vi "Flywheel At Speed Check.vi"(11 "Shooter Speed Calibration":dbl) -> ()   [LabVIEW 2016]
uses:
  Global Variables/Sensor Data.vi
  Global Variables/Shooter Calibrations.vi
  Global Variables/Robot Status.vi
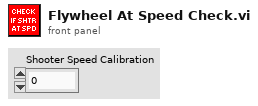
[diagram p1: front panel]
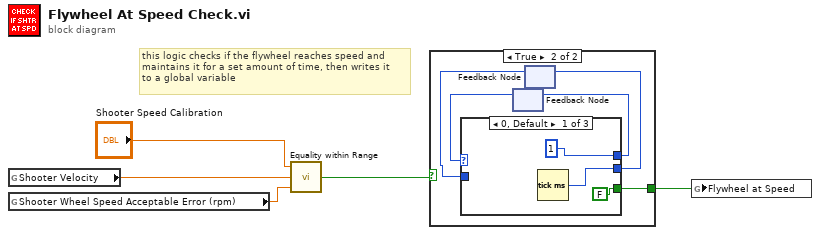
[diagram p0: block diagram]
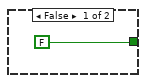
[diagram p2: hidden frame]
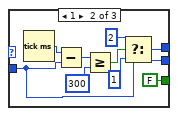
[diagram p3: hidden frame]
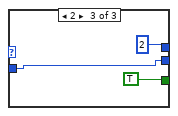
[diagram p4: hidden frame]
diagram:
  # "this logic checks if the flywheel reaches speed and\nmaintains it for a set amount of time, then writes it\nto a global variable"
  n1 = global read "Sensor Data.vi" "Shooter Velocity"() -> (w2:dbl)
  n2 = global read "Shooter Calibrations.vi" "Shooter Wheel Speed Acceptable Error (rpm)"() -> (w5:dbl)
  n3 = call "Equality within Range.vi"("Range"=w5, "Y"=w2, "X"="Shooter Speed Calibration") -> ("X = Y within Range?"=w4:bool)
  n4 = case shown="True" w4 {
    tunnel: [FALSE w7] -> w3
    frame False {
    }
    frame True {
      n5 = feedback #1() -> (w10:i32)  [unwired: 1 in]
      n6 = feedback #2() -> (w8:u32)  [unwired: 1 in]
      n7 = case shown="0, Default" w10 {
        tunnel: [1 w20 2] -> w11
        tunnel: w8 -> [_ w16 w24]
        tunnel: [w13 w16 w24] -> w9
        tunnel: [FALSE FALSE TRUE] -> w7
        frame 0, Default {
          n8 = Tick Count (ms)() -> (millisecond timer value=w13:u32)
        }
        frame 1 {
          n9 = Tick Count (ms)() -> (millisecond timer value=w23:u32)
          n10 = Subtract(x=w23, y=w16) -> (x-y=w22:u32)
          n11 = Greater Or Equal?(x=w22, y=300) -> (x >= y?=w19:bool)
          n12 = Select(t=2, s=w19, f=1) -> (s? t:f=w20:i32)
        }
        frame 2 {
        }
      }
      n13 = feedback-in #1(w11) -> ()
      n14 = feedback-in #2(w9) -> ()
    }
  }
  n15 = global write "Robot Status.vi" "Flywheel at Speed"(w3) -> ()
